vi "Enable Remote Sense.vi"(8 "error in (no error)":errorcluster, 10 "Remote Sense State (F: Disable)":bool, 11 "VISA resource name":refnum<visa-resource-name>) -> (0 "error out":errorcluster, 3 "VISA resource name out":refnum<visa-resource-name>)   [LabVIEW 2018, in "XP Power PLS600.lvlib"]
doc: "Enables (activates) or disables (de-activates) Remote Sense mode. It must be executed with On before any further remote sense commands can be execution (except for queries)."
uses:
  XP Power PLS600.lvlib
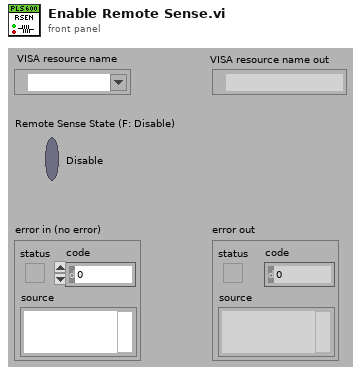
[diagram p1: front panel]
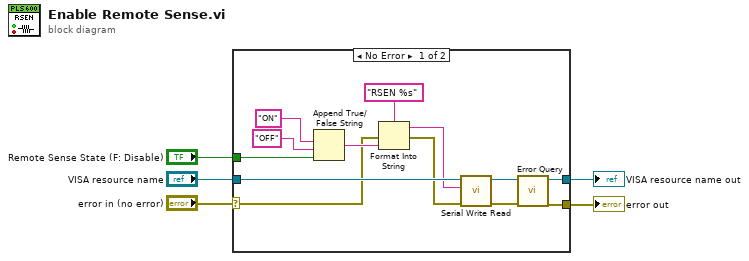
[diagram p0: block diagram]
diagram:
  n1 = case shown="No Error" "error in (no error)" {
    selector: "error in (no error)" -> [w6 w20]
    tunnel: [w18 w19] -> w5
    tunnel: [w17 w20] -> w4
    tunnel: "VISA resource name" -> [w16 w19]
    tunnel: "Remote Sense State (F: Disable)" -> [w9 _]
    frame No Error {
      n2 = Append True/False String(1:w9, 2:"OFF", 3:"ON") -> (0:w10:string)  [unwired: 1 in]
      n3 = Format Into String(format string="RSEN %s" ("Command to Send"), error in=w6, w10) -> (resulting string=w7:string, error out=w8:errorcluster)  [unwired: 1 in]
      n4 = call "Serial Write Read.vi"("error in (no error)"=w8, "Write Buffer"=w7, "VISA resource name"=w16) -> ("error out"=w14:errorcluster, "VISA resource name out"=w15:refnum<visa-resource-name>)  [unwired: 6 in, 1 out]
      n5 = call "Error Query.vi"("error in (no error)"=w14, "VISA resource name"=w15) -> ("error out"=w17:errorcluster, "VISA resource name out"=w18:refnum<visa-resource-name>)  [unwired: 6 in, 2 out]
    }
    frame Error {
    }
  }
  "VISA resource name out" <- w5
  "error out" <- w4
